vi "Array of clusters of arrays.vi"(8 "Numeric Array":dbl[](array[numeric])=[0.0, 1.0, 2.0, 3.0, 4.0], 10 "Array":cluster{"Array 2":dbl[]}[](array[cluster])=[{"Array 2"=[]}, {"Array 2"=[0.0]}, {"Array 2"=[1.0, 1.0]}, {"Array 2"=[2.0, 2.0, 2.0]}, {"Array 2"=[3.0, 3.0, 3.0, 3.0]}]) -> (0 "Numeric Array Out":dbl[](array[numeric]), 2 "Array out":cluster{"Array 2":dbl[]}[](array[cluster])=[{"Array 2"=[]}, {"Array 2"=[0.0]}, {"Array 2"=[1.0, 1.0]}, {"Array 2"=[2.0, 2.0, 2.0]}, {"Array 2"=[3.0, 3.0, 3.0, 3.0]}])   [LabVIEW 2012]
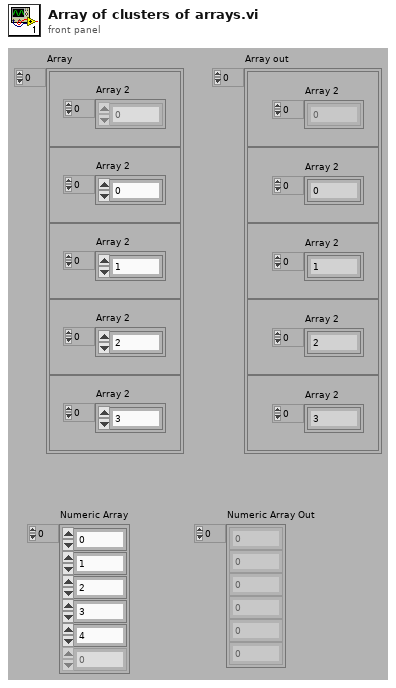
[diagram p1: front panel]
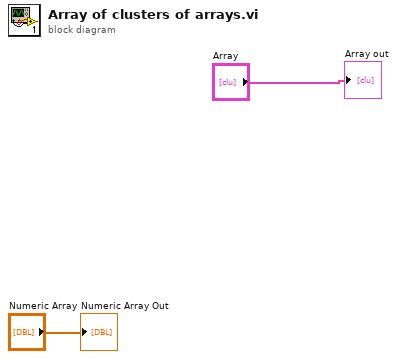
[diagram p0: block diagram]
diagram:
  "Array out" <- "Array"
  "Numeric Array Out" <- "Numeric Array"
